vi "Build Param List.vi"(1 "Topic.lvclass":refnum<class "Topic.lvclass">) -> (0 "tagged string":string)   [LabVIEW 2015, in "Topic.lvclass"]
uses:
  Topic.lvclass
  Topic.lvclass/Topic.ctl
  <vilib>/NI/Compiled HTML Menu Tool/Keyed Value Tree/Keyed Value Tree.lvclass
  XMLInterface/XmlInterface.lvclass
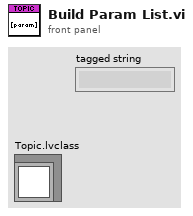
[diagram p1: front panel]
types:
  T1 = typedef "Keyed Value Tree.lvclass/Keyed Value Pair.ctl" = cluster{"Key":string, "Value":string}
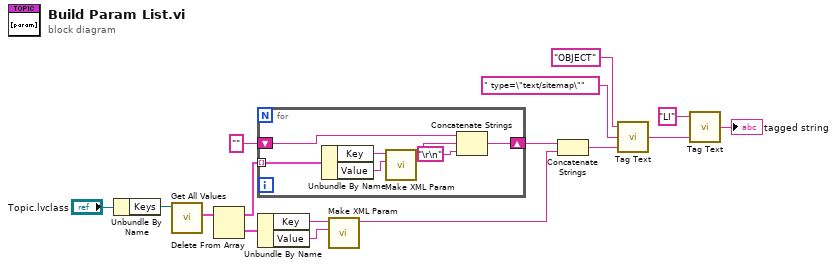
[diagram p0: block diagram]
diagram:
  n1 = Unbundle By Name("Topic.lvclass") -> ("Keys"=w5:refnum<class "Keyed Value Tree.lvclass">)
  n2 = call-dynamic "Get All Values.vi"("Keyed Value Tree in"=w5) -> ("Keyed Value Pairs"=w9:T1[])  [unwired: 8 in, 2 out]
  n3 = Delete From Array(array=w9) -> (deleted portion=w13:T1, array with subset deleted=w14:T1[])  [unwired: 2 in]
  n4 = for {
    tunnel: w14 -> [w23] mode=indexing
    shift-right: [w18] -> w16
    shift-left: "" ("Value") -> [w19]
    n5 = Unbundle By Name(w23) -> ("Key"=w22:string, "Value"=w21:string)
    n6 = call "Make XML Param.vi"("Value"=w21, "Name"=w22) -> ("param"=w20:string)  [unwired: 8 in, 1 out]
    n7 = Concatenate Strings(w19, w20, "\r\n") -> (w18:string)
  }
  n8 = Unbundle By Name(w13) -> ("Key"=w12:string, "Value"=w11:string)
  n9 = call "Make XML Param.vi"("Value"=w11, "Name"=w12) -> ("param"=w10:string)  [unwired: 8 in, 1 out]
  n10 = Concatenate Strings(w16, w10) -> (w15:string)
  n11 = call "Tag Text.vi"("Value"=w15, "properties"=" type=\"text/sitemap\"", "Tag"="OBJECT") -> ("tagged string"=w3:string)  [unwired: 2 in]
  n12 = call "Tag Text.vi"("Value"=w3, "Tag"="LI") -> ("tagged string"=→"tagged string":string)  [unwired: 3 in]
